vi "Example_TDSM.vi"(11 "Task File Name":string) -> ()   [LabVIEW 2020]
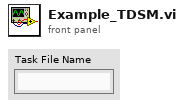
[diagram p1: front panel]
types:
  T1 = enum16{"open", "open or create", "create or replace", "create", "open (read-only)"}
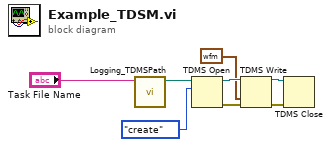
[diagram p0: block diagram]
diagram:
  n1 = call "Logging_TDMSPath.vi"("Task File Name"="Task File Name") -> ("appended path"=w4:path)  [unwired: 10 in]
  n2 = TDMS Open(10:T1."create" ("operation (0:open)"), 11:w4) -> (0:w7:errorcluster, 3:w8:refnum<k34>)  [unwired: 5 in]
  n3 = TDMS Write(0:w8, 9:waveform(dbl) {"t0"=timestamp(0 s since 1904-01-01), "dt"=1.0, "Y"=[]} ("Waveform"), 11:w7) -> (4:w6:refnum<k34>, 15:w5:errorcluster)  [unwired: 3 in, 2 out]
  n4 = TDMS Close(8:w5, 11:w6) -> ()  [unwired: 2 out]
